vi "Configure PRACH Trigger Timeout.vi"(7 "Trigger Timeout (0.1)":dbl=0.1 format="%^.3e", 8 "error in (no error)":errorcluster, 9 "Trigger Timeout Enabled (Off)":bool, 10 "Instance (1)":T1=1, 11 "VISA resource name":refnum<visa-resource-name>) -> (0 "error out":errorcluster, 3 "VISA resource name out":refnum<visa-resource-name>)   [LabVIEW 2020, in "Rohde&Schwarz CMWXP NR FR1 Measurement.lvlib"]
doc: "Selects the maximum time that the measurement waits for a trigger event before it stops in remote control mode or indicates a trigger timeout in manual operation mode. This setting has no influence on 'Free Run' measurements.\n\nAttributes:\nRSCMWXPNRFR1M_ATTR_PRACH_TRIGGER_TIMEOUT\nRSCMWXPNRFR1M_ATTR_PRACH_TRIGGER_TIMEOUT_ENABLED\n\nRemote-control command:\nTRIGger:NRSub:MEAS<i>:PRACh:TOUT"
uses:
  <instrlib>/Rohde&Schwarz CMWXP NR FR1 Measurement/Rohde&Schwarz CMWXP NR FR1 Measurement.lvlib
  <instrlib>/Rohde&Schwarz CMWXP NR FR1 Measurement/Private/_Instance.ctl
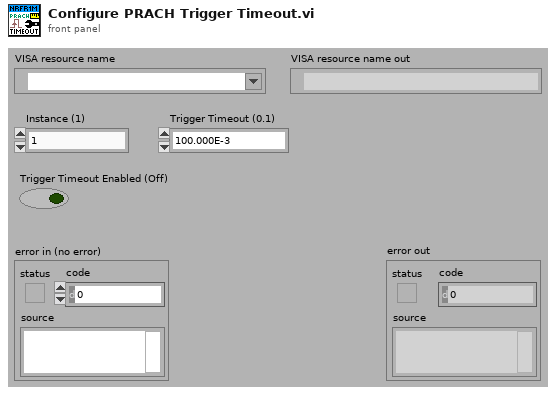
[diagram p1: front panel]
types:
  T1 = typedef "Rohde&Schwarz CMWXP NR FR1 Measurement.lvlib/_Instance.ctl" = i32
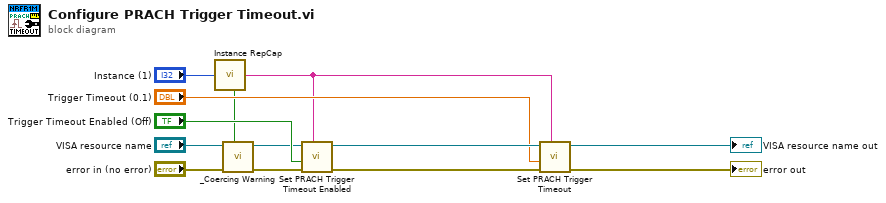
[diagram p0: block diagram]
diagram:
  n1 = call <instrlib>:"Instance RepCap.vi"("Instance In"="Instance (1)") -> ("In Range?"=w3:bool, "RepCap Identifier Out"=w2:string)  [unwired: 1 in]
  n2 = call <instrlib>:"_Coercing Warning.vi"("In Range?"=w3, "error in (no error)"="error in (no error)", "VISA resource name"="VISA resource name") -> ("error out"=w5:errorcluster, "VISA resource name out"=w1:refnum<visa-resource-name>)  [unwired: 7 in]
  n3 = call "Set PRACH Trigger Timeout Enabled"("Repeated Capabilities"=w2, "error in (no error)"=w5, "PRACH Trigger Timeout Enabled (OFF)"="Trigger Timeout Enabled (Off)", "instrument handle"=w1) -> ("error out"=w9:errorcluster, "instrument handle out"=w10:refnum<visa-resource-name>)  [unwired: 6 in]
  n4 = call "Set PRACH Trigger Timeout"("Repeated Capabilities"=w2, "error in (no error)"=w9, "PRACH Trigger Timeout (0.0)"="Trigger Timeout (0.1)", "instrument handle"=w10) -> ("error out"=→"error out":errorcluster, "instrument handle out"=→"VISA resource name out":refnum<visa-resource-name>)  [unwired: 6 in]
